vi "Write Lst_Output_Ref.vi"(8 "error in (no error)":errorcluster, 10 "Lst_Output_Ref":refnum<vi>, 11 "IOCard in":refnum<class "IOCard.lvclass">) -> (0 "error out":errorcluster, 3 "IOCard out":refnum<class "IOCard.lvclass">)   [LabVIEW 2019, in "IOCard.lvclass"]
uses:
  IOCard.lvclass
  IOCard.lvclass/IOCard.ctl
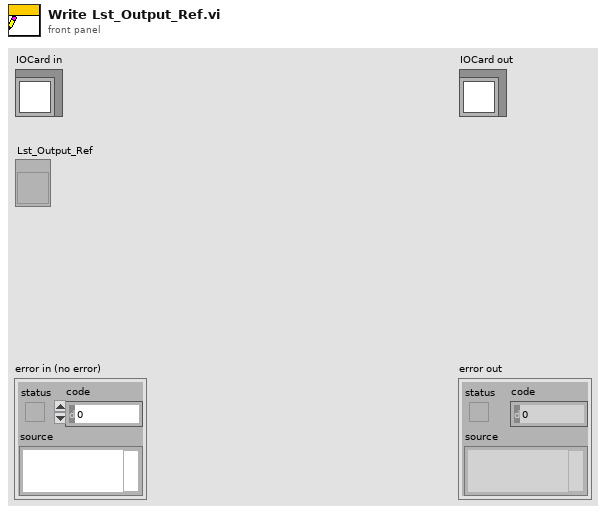
[diagram p1: front panel]
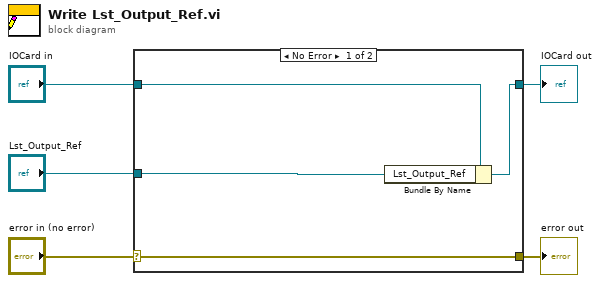
[diagram p0: block diagram]
diagram:
  n1 = case shown="No Error" "error in (no error)" {
    selector: "error in (no error)" -> [w9 w10]
    tunnel: [w9 w10] -> w4
    tunnel: [w8 w11] -> w2
    tunnel: "IOCard in" -> [w6 w11]
    tunnel: "Lst_Output_Ref" -> [w7 _]
    frame No Error {
      n2 = Bundle By Name(cluster=w6, "Lst_Output_Ref"=w7) -> (w8:refnum<class "IOCard.lvclass">)
    }
    frame Error {
    }
  }
  "error out" <- w4
  "IOCard out" <- w2
